vi "pmu_Data Conversion.vi"(0 "phasors in":csg[](array[numeric]), 1 "format":u16, 5 "freq in":sgl, 9 "dfreq in":sgl, 11 "analogs in":sgl[](array[numeric]), 12 "phasor units":u32[](array[numeric]), 13 "nominal frequency":enum16{"50 Hz", "60 Hz"}(ring)) -> (2 "analog out of range":bool, 3 "freq out of range":bool, 4 "phasor byte array":u8[](array[numeric]), 6 "freq byte array":u8[](array[numeric]), 8 "df/dt out of range":bool, 10 "dfreq byte array":u8[](array[numeric]), 14 "phasor out of range":bool, 15 "analogs byte array":u8[](array[numeric]))   [LabVIEW 2012, in "NI_EP_PMU.lvlib"]
uses:
  <vilib>/addons/Electrical Power/PMU/NI_EP_PMU.lvlib
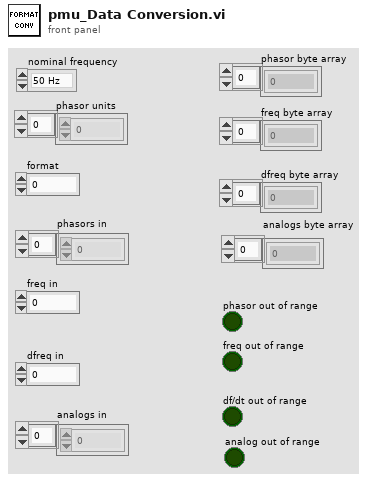
[diagram p1: front panel]
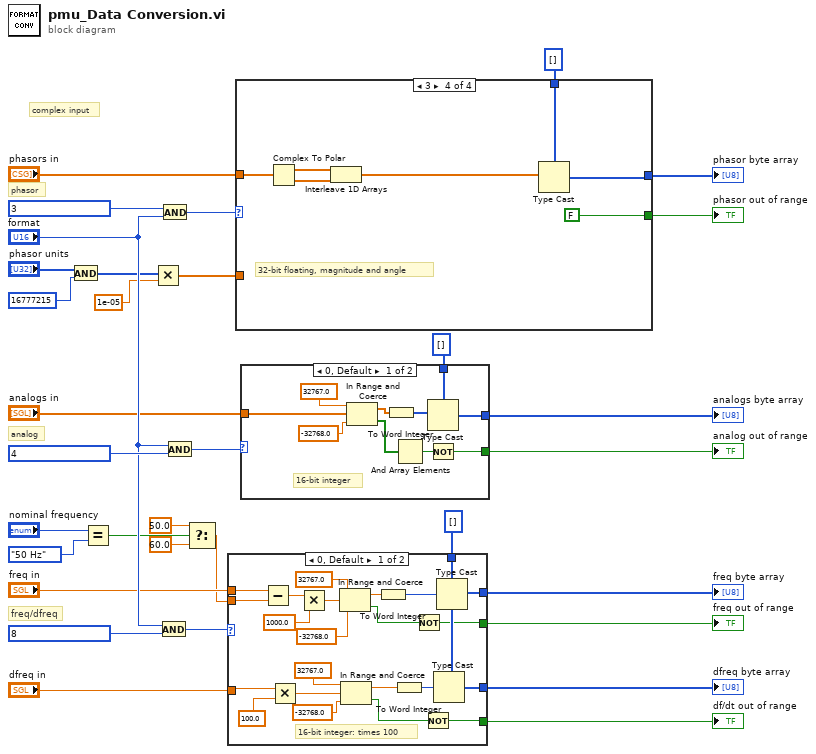
[diagram p0: block diagram]
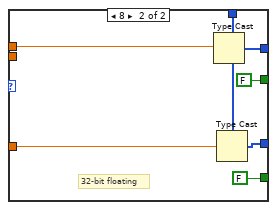
[diagram p2: hidden frame]
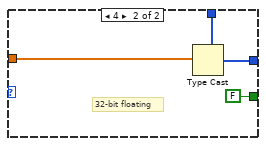
[diagram p3: hidden frame]
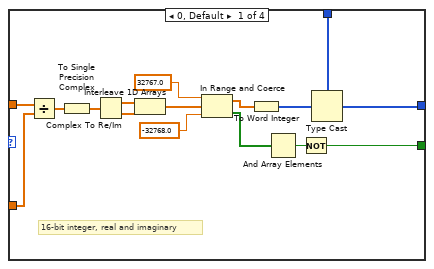
[diagram p4: hidden frame]
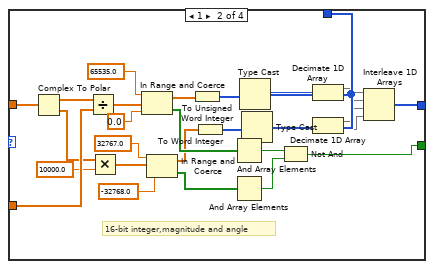
[diagram p5: hidden frame]
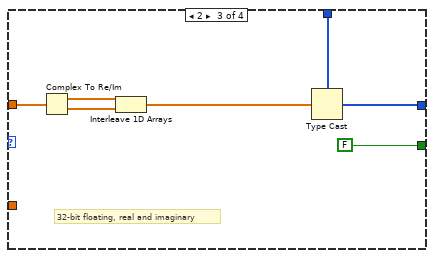
[diagram p6: hidden frame]
diagram:
  # "complex input"
  # "freq/dfreq"
  # "analog"
  # "phasor"
  n1 = And(x="phasor units", y=u32 16777215) -> (x .and. y?=w13:u32[])
  n2 = Equal?(x="nominal frequency", y=enum16{"50 Hz", "60 Hz"}."50 Hz" ("nominal frequency 2")) -> (x = y?=w7:bool)
  n3 = Multiply(x=w13, y=1e-05) -> (x*y=w11:dbl[])
  n4 = And(x="format", y=u16 8 ("x")) -> (x .and. y?=w24:u16)
  n5 = And(x=u16 3, y="format") -> (x .and. y?=w29:u16)
  n6 = And(x="format", y=u16 4 ("x")) -> (x .and. y?=w25:u16)
  n7 = Select(t=50.0, s=w7, f=60.0) -> (s? t:f=w4:dbl)
  n8 = case shown="0, Default" w24 {
    tunnel: "freq in" -> [w52 w60]
    tunnel: "dfreq in" -> [w40 w57]
    tunnel: u8[] [] ("appended array") -> [w55 w62]
    tunnel: [w56 w63] -> w17
    tunnel: [w53 w61] -> w16
    tunnel: w4 -> [w51 _]
    tunnel: [w36 FALSE] -> w3
    tunnel: [w35 FALSE] -> w2
    frame 0, Default {
      # "16-bit integer: times 100"
      n9 = Subtract(x=w52, y=w51) -> (x-y=w50:dbl)
      n10 = Multiply(x=w40, y=sgl 100.0) -> (x*y=w38:sgl)
      n11 = Multiply(x=w50, y=1000.0) -> (x*y=w48:dbl)
      n12 = In Range and Coerce(upper limit=32767.0 ("y"), x=w48, lower limit=-32768.0 ("y")) -> (coerced(x)=w45:dbl, In Range?=w37:bool)
      n13 = In Range and Coerce(upper limit=sgl 32767.0 ("y"), x=w38, lower limit=sgl -32768.0 ("y")) -> (coerced(x)=w41:sgl, In Range?=w34:bool)
      n14 = To Word Integer(number=w45) -> (16bit integer=w44:i16)
      n15 = To Word Integer(number=w41) -> (16bit integer=w54:i16)
      n16 = Not(x=w37) -> (.not. x?=w36:bool)
      n17 = Not(x=w34) -> (.not. x?=w35:bool)
      n18 = Type Cast(type=w55, x=w54) -> (*(type *) &x=w53:u8[])
      n19 = Type Cast(type=w55, x=w44) -> (*(type *) &x=w56:u8[])
    }
    frame 8 {
      # "32-bit floating"
      n20 = Type Cast(type=w62, x=w60) -> (*(type *) &x=w63:u8[])
      n21 = Type Cast(type=w62, x=w57) -> (*(type *) &x=w61:u8[])
    }
  }
  "freq byte array" <- w17
  "dfreq byte array" <- w16
  "freq out of range" <- w3
  "df/dt out of range" <- w2
  n22 = case shown="3" w29 {
    tunnel: "phasors in" -> [w74 w107 w114 w121]
    tunnel: u8[] [] ("appended array") -> [w79 w88 w110 w117]
    tunnel: [w78 w81 w109 w116] -> w26
    tunnel: w11 -> [w73 w105 _ _]
    tunnel: [w64 w80 FALSE FALSE] -> w10
    frame 0, Default {
      # "16-bit integer, real and imaginary"
      n23 = Divide(x=w74, y=w73) -> (x/y=w72:cdb[])
      n24 = To Single Precision Complex(1:w72) -> (0:w71:csg[])
      n25 = Complex To Re/Im(x + iy=w71) -> (x=w77:sgl[], y=w76:sgl[])
      n26 = Interleave 1D Arrays(w77, w76) -> (w70:sgl[])
      n27 = In Range and Coerce(upper limit=sgl 32767.0, x=w70, lower limit=sgl -32768.0) -> (coerced(x)=w67:sgl[], In Range?=w66:bool[])
      n28 = To Word Integer(number=w67) -> (16bit integer=w75:i16[])
      n29 = And Array Elements(Boolean array=w66) -> (logical AND=w65:bool)
      n30 = Not(x=w65) -> (.not. x?=w64:bool)
      n31 = Type Cast(type=w79, x=w75) -> (*(type *) &x=w78:u8[])
    }
    frame 1 {
      # "16-bit integer,magnitude and angle"
      n32 = Complex To Polar(r * e^(i*theta)=w107) -> (r=w106:sgl[], theta=w104:sgl[])
      n33 = Divide(x=w106, y=w105) -> (x/y=w102:dbl[])
      n34 = Multiply(x=w104, y=sgl 10000.0) -> (x*y=w99:sgl[])
      n35 = In Range and Coerce(upper limit=65535.0, x=w102, lower limit=0.0) -> (coerced(x)=w93:dbl[], In Range?=w96:bool[])
      n36 = In Range and Coerce(upper limit=sgl 32767.0, x=w99, lower limit=sgl -32768.0) -> (coerced(x)=w92:sgl[], In Range?=w90:bool[])
      n37 = To Unsigned Word Integer(number=w93) -> (unsigned 16bit integer=w91:u16[])
      n38 = To Word Integer(number=w92) -> (16bit integer=w89:i16[])
      n39 = And Array Elements(Boolean array=w96) -> (logical AND=w95:bool)
      n40 = And Array Elements(Boolean array=w90) -> (logical AND=w94:bool)
      n41 = Type Cast(type=w88, x=w91) -> (*(type *) &x=w87:u8[])
      n42 = Type Cast(type=w88, x=w89) -> (*(type *) &x=w86:u8[])
      n43 = Not And(1:w94, 2:w95) -> (0:w80:bool)
      n44 = Decimate 1D Array(w87) -> (w85:u8[], w84:u8[])
      n45 = Decimate 1D Array(w86) -> (w83:u8[], w82:u8[])
      n46 = Interleave 1D Arrays(w85, w84, w83, w82) -> (w81:u8[])
    }
    frame 2 {
      # "32-bit floating, real and imaginary"
      n47 = Complex To Re/Im(x + iy=w114) -> (x=w113:sgl[], y=w112:sgl[])
      n48 = Interleave 1D Arrays(w113, w112) -> (w111:sgl[])
      n49 = Type Cast(type=w110, x=w111) -> (*(type *) &x=w109:u8[])
    }
    frame 3 {
      # "32-bit floating, magnitude and angle"
      n50 = Complex To Polar(r * e^(i*theta)=w121) -> (r=w120:sgl[], theta=w119:sgl[])
      n51 = Interleave 1D Arrays(w120, w119) -> (w118:sgl[])
      n52 = Type Cast(type=w117, x=w118) -> (*(type *) &x=w116:u8[])
    }
  }
  "phasor byte array" <- w26
  "phasor out of range" <- w10
  n53 = case shown="0, Default" w25 {
    tunnel: "analogs in" -> [w126 w134]
    tunnel: u8[] [] ("appended array") -> [w130 w135]
    tunnel: [w129 w133] -> w21
    tunnel: [w122 FALSE] -> w1
    frame 0, Default {
      # "16-bit integer"
      n54 = In Range and Coerce(upper limit=sgl 32767.0 ("y"), x=w126, lower limit=sgl -32768.0 ("y")) -> (coerced(x)=w125:sgl[], In Range?=w123:bool[])
      n55 = To Word Integer(number=w125) -> (16bit integer=w131:i16[])
      n56 = And Array Elements(Boolean array=w123) -> (logical AND=w124:bool)
      n57 = Type Cast(type=w130, x=w131) -> (*(type *) &x=w129:u8[])
      n58 = Not(x=w124) -> (.not. x?=w122:bool)
    }
    frame 4 {
      # "32-bit floating"
      n59 = Type Cast(type=w135, x=w134) -> (*(type *) &x=w133:u8[])
    }
  }
  "analogs byte array" <- w21
  "analog out of range" <- w1
